vi "Error Query.vi"(8 "error in (no error)":errorcluster, 11 "VISA resource name":refnum<visa-resource-name>) -> (0 "error out":errorcluster, 1 "Error Message":string, 2 "Error Code":i32[](array[numeric]), 3 "VISA resource name out":refnum<visa-resource-name>)   [LabVIEW 2014, in "Agilent ESA PSA Series.lvlib"]
doc: "Queries the instrument for any errors in the instrument's error queue. It will continue to read errors until all errors have been read from the instrument. Any errors will be returned in the <B>error out</B> control.\n\n<B>Note:</B>\n\nThis VI is called automatically by most driver VIs so it is not usually necessary to call this in an application."
uses:
  Agilent ESA PSA Series.lvlib
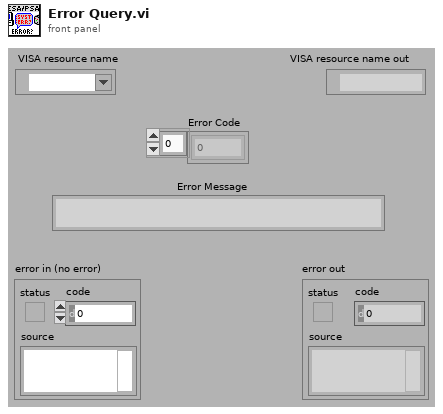
[diagram p1: front panel]
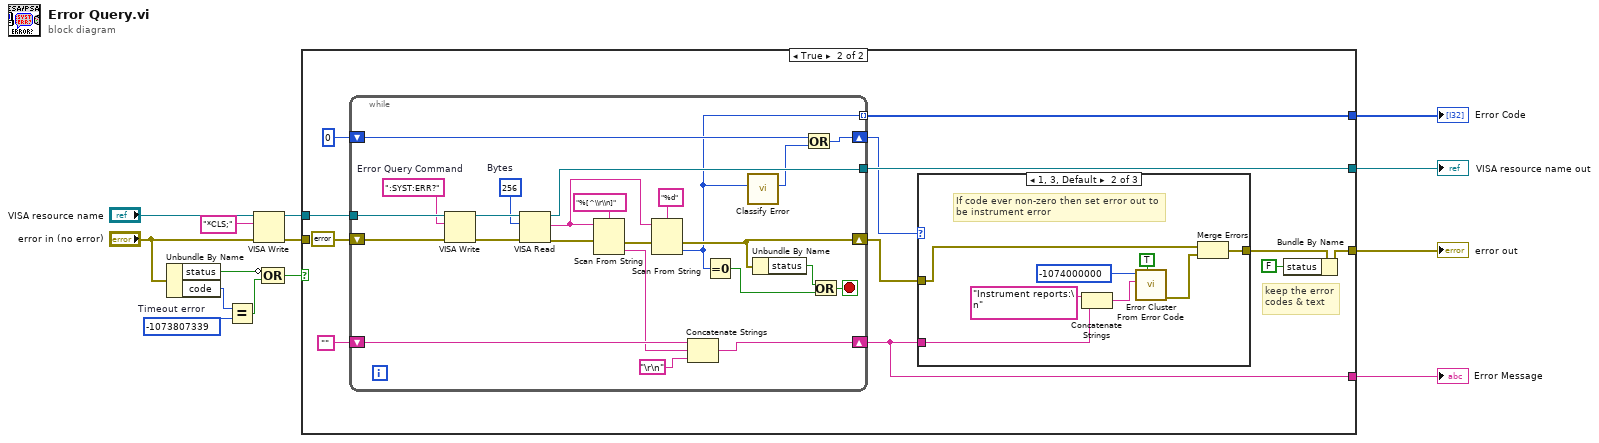
[diagram p0: block diagram]
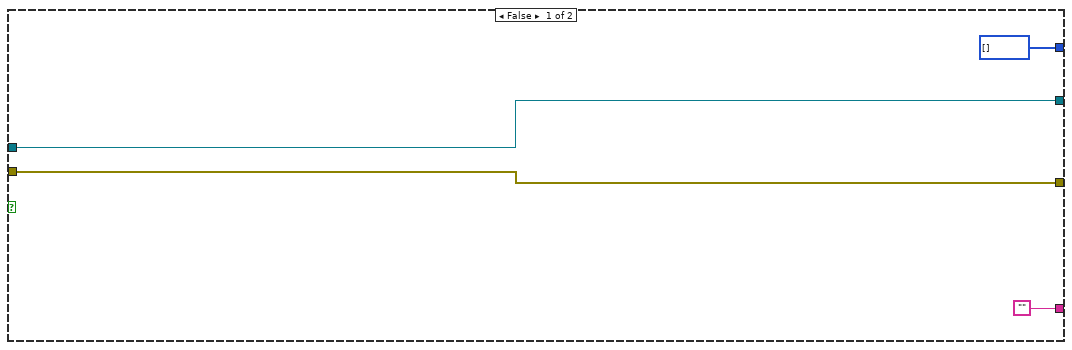
[diagram p2: hidden frame]
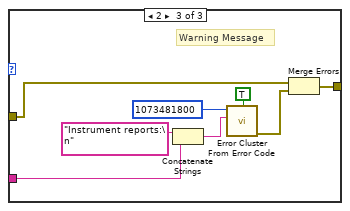
[diagram p4: hidden frame]
diagram:
  w11 = -1073807339  # Timeout error
  n1 = Unbundle By Name("error in (no error)") -> ("status"=w12:bool, "code"=w9:i32)
  n2 = Equal?(x=w9, y=w11) -> (x = y?=w10:bool)
  n3 = VISA Write(VISA resource name="VISA resource name", write buffer="*CLS;", error in (no error)="error in (no error)") -> (VISA resource name out=w3:refnum<visa-resource-name>, error out=w2:errorcluster)  [unwired: 1 out]
  n4 = Compound Arithmetic op=OR(invert w12, w10) -> (w8:bool)
  n5 = case shown="True" w8 {
    tunnel: [w18 w30] -> w14
    tunnel: w3 -> [w18 w29]
    tunnel: w2 -> [w17 _]
    tunnel: [w17 w20] -> w13
    tunnel: ["" w26] -> w7
    tunnel: [i32[] [] w25] -> w6
    frame False {
    }
    frame True {
      # "keep the error\ncodes & text"
      n6 = while {
        tunnel: [w71] -> w30
        tunnel: w29 -> [w70]
        shift-right: [w58] -> w26
        shift-left: "" -> [w61]
        shift-right: [w52] -> w23
        shift-left: i16 0 -> [w51]
        shift-right: [w56] -> w24
        shift-left: errorcluster {"status"=FALSE, "code"=0, "source"=""} ("error IO") -> [w57]
        tunnel: [w49] -> w25 mode=indexing
        stop <- w64 stop-if-true
        w68 = u32 256  # Bytes
        w66 = ":SYST:ERR?"  # Error Query Command
        n7 = VISA Write(VISA resource name=w70, write buffer=w66, error in (no error)=w57) -> (VISA resource name out=w69:refnum<visa-resource-name>, error out=w67:errorcluster)  [unwired: 1 out]
        n8 = VISA Read(VISA resource name=w69, byte count=w68, error in (no error)=w67) -> (VISA resource name out=w71:refnum<visa-resource-name>, read buffer=w62:string, error out=w55:errorcluster)  [unwired: 1 out]
        n9 = Scan From String(format string="%[^\\r\\n]", input string=w62, error in=w55) -> (error out=w54:errorcluster, output 1=w59:string)  [unwired: 2 in, 2 out]
        n10 = Scan From String(format string="%d", input string=w62, error in=w54) -> (error out=w56:errorcluster, output 1=w49:i32)  [unwired: 2 in, 2 out]
        n11 = Concatenate Strings(w61, w59, "\r\n") -> (w58:string)
        n12 = Equal To 0?(x=w49) -> (x = 0?=w50:bool)
        n13 = call "Classify Error.vi"("Error Code"=w49) -> ("Error Classification"=w48:u32)  [unwired: 10 in]
        n14 = Unbundle By Name(w56) -> ("status"=w53:bool)
        n15 = Or(x=w51, y=w48) -> (x .or. y?=w52:u32)
        n16 = Or(x=w53, y=w50) -> (x .or. y?=w64:bool)
      }
      n17 = case shown="1, 3, Default" w23 {
        tunnel: w26 -> [_ w38 w46]
        tunnel: [w31 w32 w41] -> w22
        tunnel: w24 -> [w31 w33 w42]
        frame 0 {
        }
        frame 1, 3, Default {
          # "If code ever non-zero then set error out to\nbe instrument error"
          n18 = Concatenate Strings("Instrument reports:\n" ("Source"), w38) -> (w36:string)
          n19 = call "Error Cluster From Error Code.vi"("show call chain? (False)"=TRUE, "error message (\"\")"=w36, "error code (0)"=-1074000000 ("Code")) -> ("error out"=w34:errorcluster)  [unwired: 6 in]
          n20 = Merge Errors(w33, w34) -> (w32:errorcluster)
        }
        frame 2 {
          # "Warning Message"
          n21 = Concatenate Strings("Instrument reports:\n" ("Source"), w46) -> (w44:string)
          n22 = call "Error Cluster From Error Code.vi"("is warning? (False)"=TRUE ("show call chain? (False)"), "error message (\"\")"=w44, "error code (0)"=1073481800 ("Code")) -> ("error out"=w43:errorcluster)  [unwired: 6 in]
          n23 = Merge Errors(w42, w43) -> (w41:errorcluster)
        }
      }
      n24 = Bundle By Name(cluster=w22, "status"=FALSE) -> (w20:errorcluster)
    }
  }
  "VISA resource name out" <- w14
  "error out" <- w13
  "Error Message" <- w7
  "Error Code" <- w6
